vi "Write Pressure Valve Opening (%).vi"(10 "Pressure Valve Opening (%)":dbl=2.0, 11 "PressureValve in":refnum<class "PressureValve.lvclass">) -> (3 "PressureValve out":refnum<class "PressureValve.lvclass">)   [LabVIEW 2015, in "PressureValve.lvlib" / "PressureValve.lvclass"]
uses:
  <userlib>/Common/Devices/PressureValve/PressureValve/PressureValve.lvclass
  <userlib>/Common/Devices/PressureValve/PressureValve/PressureValve.lvclass/PressureValve.ctl
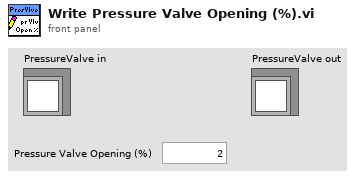
[diagram p1: front panel]
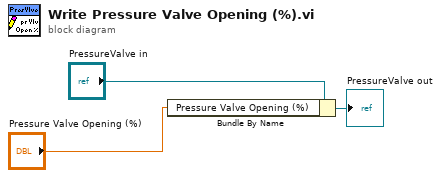
[diagram p0: block diagram]
diagram:
  n1 = Bundle By Name(cluster="PressureValve in", "Pressure Valve Opening (%)"="Pressure Valve Opening (%)") -> (→"PressureValve out":refnum<class "PressureValve.lvclass">)
